vi "Log file.vi"(8 "error in (no error)":errorcluster, 10 "Logging Data":T2, 11 "Car Wash Controller Actor in":refnum<class "Car Wash Controller Actor.lvclass">) -> (0 "error out":errorcluster, 3 "Car Wash Controller Actor out":refnum<class "Car Wash Controller Actor.lvclass">)   [LabVIEW 2019, in "Car Wash Controller Actor.lvlib" / "Car Wash Controller Actor.lvclass"]
uses:
  Car Wash Controller Actor.lvclass
  Error Levels.ctl
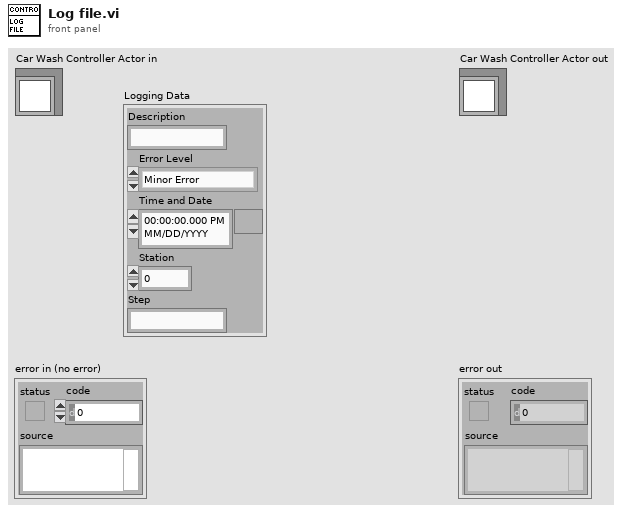
[diagram p1: front panel]
types:
  T1 = typedef "Car Wash Controller Actor.lvlib/Car Wash Controller Actor.lvclass/Error Levels.ctl" = enum16{"Minor Error", "Wash Cycle Error", "System Error"}
  T2 = cluster{"Description":string, "Error Level":T1, "Time and Date":timestamp, "Station":u32, "Step":string}
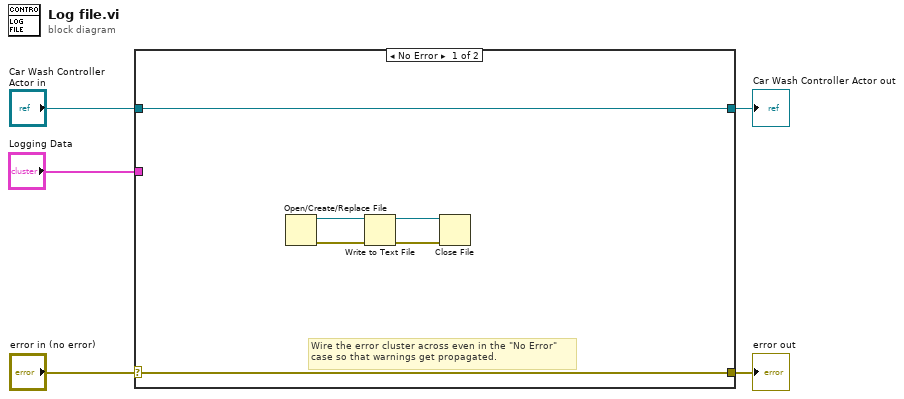
[diagram p0: block diagram]
diagram:
  n1 = case shown="No Error" "error in (no error)" {
    selector: "error in (no error)" -> [w10 w13]
    tunnel: [w10 w13] -> w4
    tunnel: [w11 w12] -> w2
    tunnel: "Car Wash Controller Actor in" -> [w11 w12]
    tunnel: "Logging Data" -> [_ _]
    frame No Error {
      # "Wire the error cluster across even in the \"No Error\"\ncase so that warnings get propagated."
      n2 = Open/Create/Replace File() -> (refnum out=w9:refnum<file>, error out=w8:errorcluster)  [unwired: 6 in, 1 out]
      n3 = Write to Text File(file (use dialog)=w9, error in=w8) -> (refnum out=w6:refnum<file>, error out=w7:errorcluster)  [unwired: 2 in, 1 out]
      n4 = Close File(refnum=w6, error in=w7) -> ()  [unwired: 2 out]
    }
    frame Error {
    }
  }
  "error out" <- w4
  "Car Wash Controller Actor out" <- w2
